vi "setLaserParameter.vi"(6 "SetLaserEnergy":dbl(slide) scale=0.0..20.0, 7 "频率/Hz":u8=60, 8 "error in (no error)":errorcluster, 9 "LaserHV":u8, 10 "LaserQuantity":u16, 11 "VISA resource name":refnum<visa-resource-name>) -> (0 "error out":errorcluster)   [LabVIEW 2013]
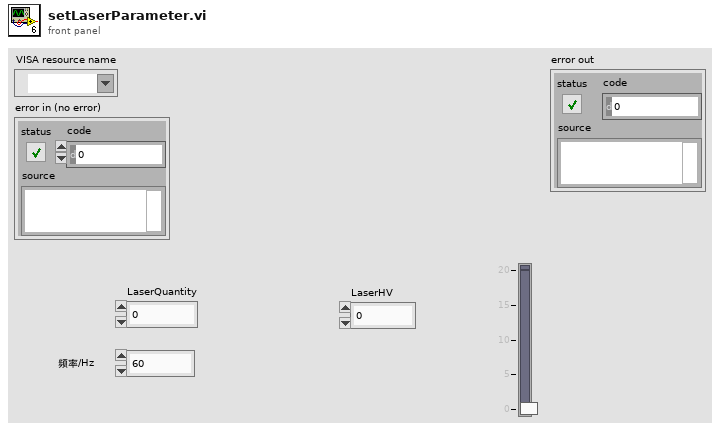
[diagram p1: front panel]
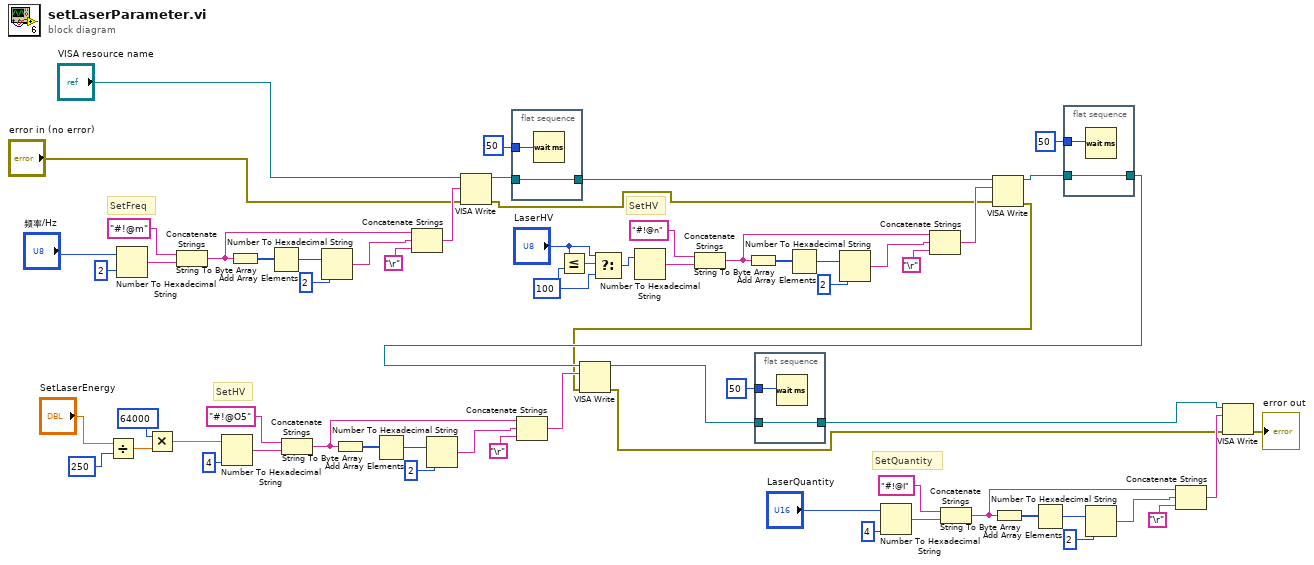
[diagram p0: block diagram]
diagram:
  w53 = u8 100 ("y")
  # "SetQuantity"
  # "SetHV"
  # "SetHV"
  # "SetFreq"
  n1 = Divide(x="SetLaserEnergy", y=250) -> (x/y=w28:dbl)
  n2 = Number To Hexadecimal String(1:i16 2 ("width (-)"), 2:"频率/Hz") -> (0:w63:string)
  n3 = Multiply(x=64000, y=w28) -> (x*y=w26:dbl)
  n4 = Concatenate Strings("#!@m" ("string"), w63) -> (w59:string)
  n5 = Number To Hexadecimal String(1:i16 4 ("width (-)"), 2:w26) -> (0:w36:string)
  n6 = String To Byte Array(string=w59) -> (unsigned byte array=w62:u8[])
  n7 = Add Array Elements(numeric array=w62) -> (sum=w61:u8)
  n8 = Concatenate Strings("#!@O5" ("string"), w36) -> (w32:string)
  n9 = Number To Hexadecimal String(1:i16 2 ("width (-)"), 2:w61) -> (0:w58:string)
  n10 = String To Byte Array(string=w32) -> (unsigned byte array=w35:u8[])
  n11 = Add Array Elements(numeric array=w35) -> (sum=w34:u8)
  n12 = Concatenate Strings(w59, w58, "\r") -> (w56:string)
  n13 = Number To Hexadecimal String(1:i16 2 ("width (-)"), 2:w34) -> (0:w31:string)
  n14 = VISA Write(VISA resource name="VISA resource name", write buffer=w56, error in (no error)="error in (no error)") -> (VISA resource name out=w42:refnum<visa-resource-name>, error out=w4:errorcluster)  [unwired: 1 out]
  n15 = flat-sequence {
    tunnel: w42 -> [w66]
    tunnel: [w66] -> w41
    tunnel: u32 50 ("delay before read (ms)") -> [w67]
    frame #0 {
      n16 = Wait (ms)(milliseconds to wait=w67) -> ()  [unwired: 1 out]
    }
  }
  n17 = Concatenate Strings(w32, w31, "\r") -> (w24:string)
  n18 = Less Or Equal?(x="LaserHV", y=w53) -> (x <= y?=w55:bool)
  n19 = Select(t="LaserHV", s=w55, f=w53) -> (s? t:f=w44:u8)
  n20 = Number To Hexadecimal String(2:w44) -> (0:w51:string)  [unwired: 1 in]
  n21 = Concatenate Strings("#!@n" ("string"), w51) -> (w47:string)
  n22 = String To Byte Array(string=w47) -> (unsigned byte array=w50:u8[])
  n23 = flat-sequence {
    tunnel: w11 -> [w69]
    tunnel: [w69] -> w10
    tunnel: u32 50 ("delay before read (ms)") -> [w68]
    frame #0 {
      n24 = Wait (ms)(milliseconds to wait=w68) -> ()  [unwired: 1 out]
    }
  }
  n25 = Add Array Elements(numeric array=w50) -> (sum=w49:u8)
  n26 = Number To Hexadecimal String(1:i16 2 ("width (-)"), 2:w49) -> (0:w46:string)
  n27 = Number To Hexadecimal String(1:i16 4 ("width (-)"), 2:"LaserQuantity") -> (0:w21:string)
  n28 = Concatenate Strings(w47, w46, "\r") -> (w40:string)
  n29 = Concatenate Strings("#!@I" ("string"), w21) -> (w17:string)
  n30 = VISA Write(VISA resource name=w41, write buffer=w40, error in (no error)=w4) -> (VISA resource name out=w39:refnum<visa-resource-name>, error out=w3:errorcluster)  [unwired: 1 out]
  n31 = VISA Write(VISA resource name=w23, write buffer=w24, error in (no error)=w3) -> (VISA resource name out=w11:refnum<visa-resource-name>, error out=w2:errorcluster)  [unwired: 1 out]
  n32 = String To Byte Array(string=w17) -> (unsigned byte array=w20:u8[])
  n33 = Add Array Elements(numeric array=w20) -> (sum=w19:u8)
  n34 = flat-sequence {
    tunnel: w39 -> [w71]
    tunnel: [w71] -> w23
    tunnel: u32 50 ("delay before read (ms)") -> [w70]
    frame #0 {
      n35 = Wait (ms)(milliseconds to wait=w70) -> ()  [unwired: 1 out]
    }
  }
  n36 = Number To Hexadecimal String(1:i16 2 ("width (-)"), 2:w19) -> (0:w16:string)
  n37 = Concatenate Strings(w17, w16, "\r") -> (w9:string)
  n38 = VISA Write(VISA resource name=w10, write buffer=w9, error in (no error)=w2) -> (error out=→"error out":errorcluster)  [unwired: 2 out]
